vi "Test_scan-from-string.vi"() -> ()   [LabVIEW 2012]
panel:
  out "Array":string[](array[string])
  in  "stop":bool
  out "output 3":string
  in  "format string":string
  in  "input string":string
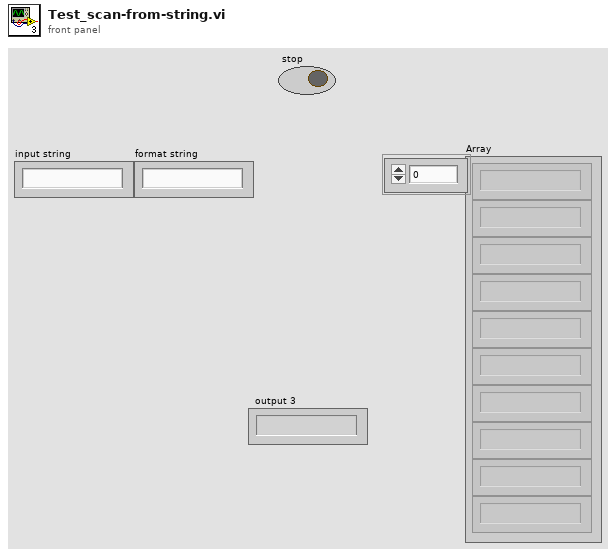
[diagram p1: front panel]
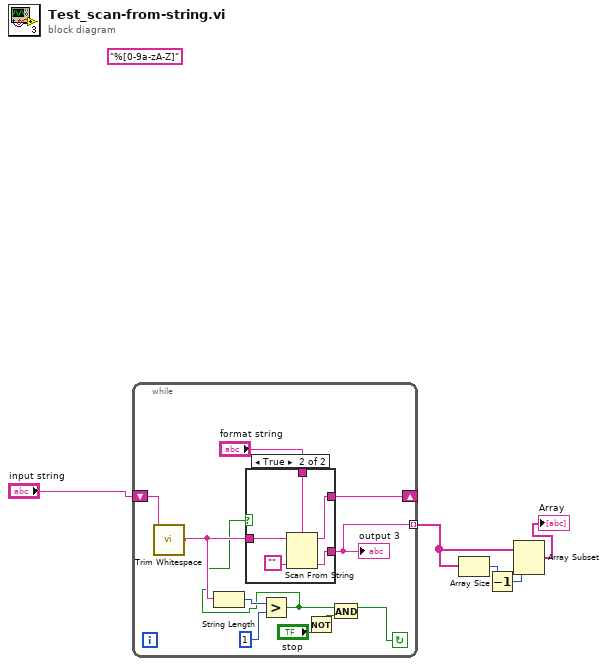
[diagram p0: block diagram]
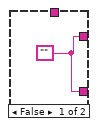
[diagram p2: hidden frame]
diagram:
  (unwired) "%[0-9a-zA-Z]" ("format string")
  n1 = while {
    shift-right: [w15] -> _
    shift-left: "input string" -> [w16]
    tunnel: [w7] -> w2 mode=indexing
    stop <- w11 continue-if-true
    n2 = call <vilib>:"Trim Whitespace.vi"("string"=w16) -> ("trimmed string"=w14:string)  [unwired: 1 in]
    n3 = String Length(string=w14) -> (length=w13:i32)
    n4 = Greater?(x=w13, y=1) -> (0:w6:bool)
    n5 = case shown="True" w6 {
      tunnel: [w17 w22] -> w15
      tunnel: w14 -> [_ w21]
      tunnel: "format string" -> [_ w20]
      tunnel: [w17 w19] -> w7
      frame False {
        w17 = ""
      }
      frame True {
        n6 = Scan From String(format string=w20, input string=w21, default 1="") -> (remaining string=w22:string, output 1=w19:string)  [unwired: 2 in, 2 out]
      }
    }
    "output 3" <- w7
    n7 = Not(x="stop") -> (.not. x?=w9:bool)
    n8 = And(x=w6, y=w9) -> (x .and. y?=w11:bool)
  }
  n9 = Array Size(array=w2) -> (size(s)=w4:i32)
  n10 = Decrement(x=w4) -> (x-1=w3:i32)
  n11 = Array Subset(array=w2, length=w3) -> (→"Array":string[])  [unwired: 1 in]
